vi "Test 1.vi"(8 "error in (no error)":errorcluster, 11 "Test Case In":refnum<class "Day 11 Test.lvclass">) -> (0 "error out":errorcluster, 3 "Test Case Out":refnum<class "Day 11 Test.lvclass">)   [LabVIEW 2020, in "Day 11 Test.lvclass"]
uses:
  Day 11 Test.lvclass
  Day 11 Test.lvclass/Day 11 Test.ctl
  4993e8ee-a06a-463a-9684-69129f64d5ce.vi
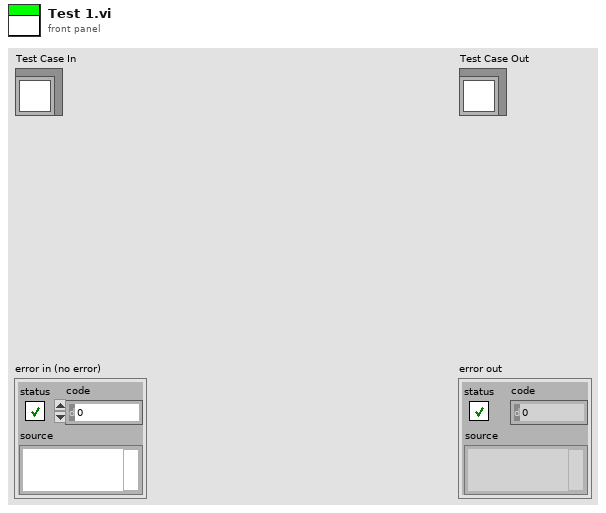
[diagram p1: front panel]
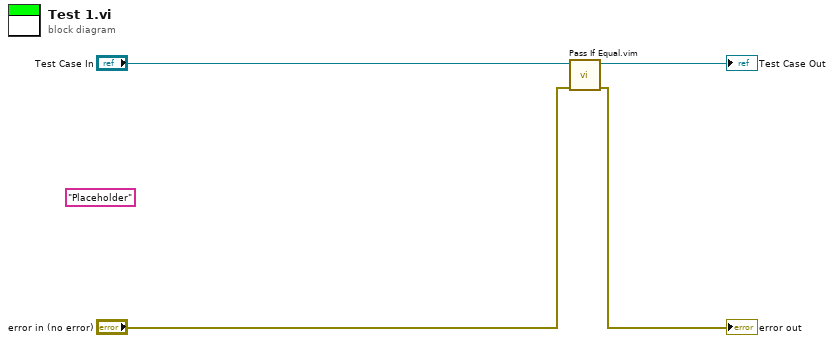
[diagram p0: block diagram]
diagram:
  (unwired) "Placeholder"
  n1 = call "Pass If Equal.vim"("error in (no error)"="error in (no error)", "LUnit Test Case In"="Test Case In") -> ("error out"=→"error out":errorcluster, "LUnit Test Case Out"=→"Test Case Out":refnum<class "Day 11 Test.lvclass">)  [unwired: 8 in]
